vi "PicoScope9400_Example.vi"() -> ()   [LabVIEW 2020]
panel:
  in  "PicoSample4.ICOMRC":refnum<k7>
  out "Plot":cluster{"Xorig":sgl, "Xint":sgl, "Array":sgl[]}(graph)
  in  "Data":bool
  in  "Run":bool
  in  "Stop":bool
  in  "Single":bool
  in  "Command":string
  in  "ON":bool
  out "Response":string
  out "error out":errorcluster
  in  "Send":bool
  in  "OFF":bool
  in  "error in":errorcluster
  # "This VI demostrates the basic steps needed to create Active X client in LabVIEW"
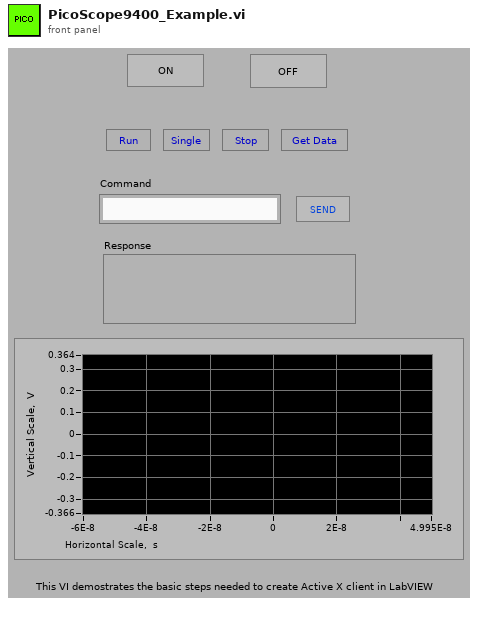
[diagram p1: front panel]
types:
  T1 = cluster{"Xmin":sgl, "Xint":sgl, "Data Array":sgl[]}
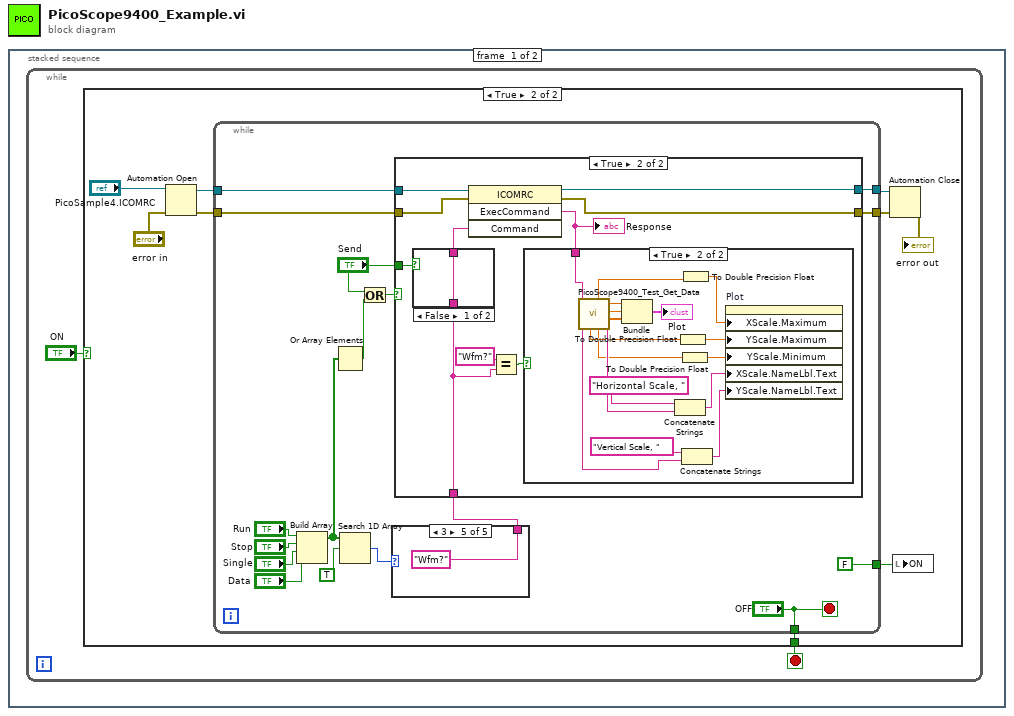
[diagram p0: block diagram]
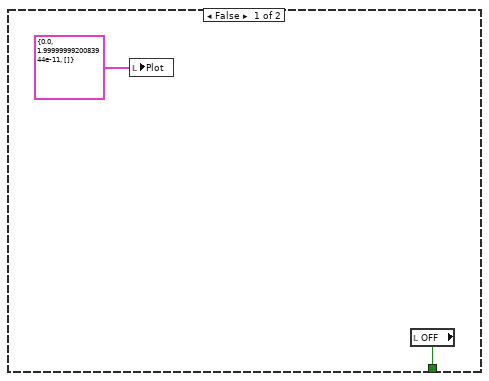
[diagram p2: hidden frame]
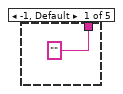
[diagram p3: hidden frame]
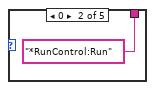
[diagram p4: hidden frame]
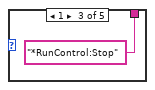
[diagram p5: hidden frame]
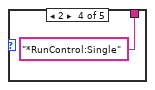
[diagram p6: hidden frame]
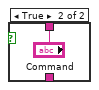
[diagram p9: hidden frame]
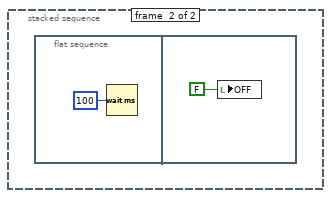
[diagram p10: hidden frame]
diagram:
  n1 = stacked-sequence {
    frame #0 {
      n2 = while {
        stop <- w2 stop-if-true
        n3 = case shown="True" "ON" {
          tunnel: [w3 w7] -> w2
          frame False {
            n4 = local write "Plot"(cluster{"Xorig":sgl, "Xint":sgl, "Array":sgl[]} {"Xorig"=0.0, "Xint"=2e-11, "Array"=[]} ("Single Plot")) -> ()
            n5 = local read "OFF"() -> (w3:bool)
          }
          frame True {
            n6 = Automation Open(error in (no error)="error in", Automation Refnum="PicoSample4.ICOMRC") -> (Automation Refnum=w12:refnum<k7>, error out=w11:errorcluster)  [unwired: 2 in]
            n7 = while {
              tunnel: w12 -> [w30]
              tunnel: w11 -> [w29]
              tunnel: [w28] -> w10
              tunnel: [w27] -> w9
              tunnel: ["OFF"] -> w7
              tunnel: [FALSE] -> w6
              stop <- "OFF" stop-if-true
              n8 = Build Array("Run", "Stop", "Single", "Data") -> (w19:bool[])
              n9 = Or Array Elements(Boolean array=w19) -> (logical OR=w18:bool)
              n10 = Search 1D Array(1D array=w19, element=TRUE) -> (index of element=w15:i32)  [unwired: 1 in]
              n11 = Or(x="Send", y=w18) -> (x .or. y?=w20:bool)
              n12 = case shown="3" w15 {
                tunnel: ["" "*RunControl:Run" "*RunControl:Stop" "*RunControl:Single" "Wfm?"] -> w14
                frame -1, Default {
                }
                frame 0 {
                }
                frame 1 {
                }
                frame 2 {
                }
                frame 3 {
                }
              }
              n13 = case shown="True" w20 {
                tunnel: w30 -> [w37 w47]
                tunnel: w29 -> [w36 w46]
                tunnel: [w37 w45] -> w28
                tunnel: [w36 w44] -> w27
                tunnel: w14 -> [_ w40]
                tunnel: "Send" -> [_ w42]
                frame False {
                }
                frame True {
                  n14 = case shown="False" w42 {
                    tunnel: [w65 "Command"] -> w43
                    tunnel: w40 -> [w65 _]
                    frame False {
                    }
                    frame True {
                    }
                  }
                  n15 = invoke class="ICOMRC" method="ExecCommand"(reference=w47, error in=w46, "Command"=w43) -> (reference out=w45:refnum<k7>, error out=w44:errorcluster, "ExecCommand"=w38:string)  [unwired: 1 in, 1 out]
                  "Response" <- w38
                  n16 = Equal?(x="Wfm?", y=w40) -> (x = y?=w41:bool)
                  n17 = case shown="True" w41 {
                    tunnel: w38 -> [_ w64]
                    frame False {
                    }
                    frame True {
                      n18 = call "PicoScope9400_Test_Get_Data.vi"("ExecCommand"=w64) -> ("XU"=w62:string, "Data Array"=w57:sgl[], "Xint"=w56:sgl, "Xmin"=w48:sgl, "Ymin"=w49:sgl, "Xmax"=w50:sgl, "Ymax"=w51:sgl, "YU"=w59:string)  [unwired: 2 in, 1 out]
                      n19 = Bundle("Xmin"=w48, "Xint"=w56, "Data Array"=w57) -> (→"Plot":T1)  [unwired: 1 in]
                      n20 = Concatenate Strings("Horizontal Scale, " ("string"), w62) -> (w61:string)
                      n21 = To Double Precision Float(number=w51) -> (double precision float=w52:dbl)
                      n22 = To Double Precision Float(number=w49) -> (double precision float=w53:dbl)
                      n23 = To Double Precision Float(number=w50) -> (double precision float=w54:dbl)
                      n24 = Concatenate Strings("Vertical Scale, " ("string"), w59) -> (w58:string)
                      n25 = property on="Plot" class="WFGraph (strict)"("XScale.Maximum"=w54, "YScale.Maximum"=w52, "YScale.Minimum"=w53, "XScale.NameLbl.Text"=w61, "YScale.NameLbl.Text"=w58) -> ()  [unwired: 2 in, 2 out]
                    }
                  }
                }
              }
            }
            n26 = Automation Close(3:w9, 5:w10) -> (0:→"error out":errorcluster)
            n27 = local write "ON"(w6) -> ()
          }
        }
      }
    }
    frame #1 {
      n28 = flat-sequence {
        frame #0 {
          n29 = Wait (ms)(milliseconds to wait=u32 100) -> ()  [unwired: 1 out]
        }
        frame #1 {
          n30 = local write "OFF"(FALSE ("stop")) -> ()
        }
      }
    }
  }
